vi "Export Origin - IV.vi"(8 "Error In":errorcluster, 9 "Workspace":path, 10 "Session properties":T4, 11 "IV measurement":T1={"Name"="", "Comment"="", "Time"=timestamp(0 s since 1904-01-01), "Folder"=path "", "IV properties"={"T"=0.0, "Vstart"=-0.5, "Vstop"=0.5, "Vpoints"=10.0, "Settling"=0.01, "I limit"=0.1, "Log mapping"=FALSE, "Averaging"=0.0}, "GUID"=""} {"IV properties"."Settling" min=0.0 max=65535.0}) -> (0 "Error Out":errorcluster)   [LabVIEW 2019]
doc: "Handles export of a I-V measurement to an Origin project, displays a GUI window"
uses:
  Type defs/Session properties Type Def.ctl
  Type defs/IV measurement Type Def.ctl
  Type defs/IV properties Type Def.ctl
  <vilib>/Utility/sysdir.llb/System Directory Type.ctl
panel:
  in  "Comment":T3(array[ring])=[enum."Temperature"] caption="Parameters to be placed in comments"
  in  "Save and exit after export":bool
  in  "Export to current Origin instance":bool
  out "String":string
  in  "Path":path caption="Export file as:"
  in  "Export":bool
  in  "Cancel":bool
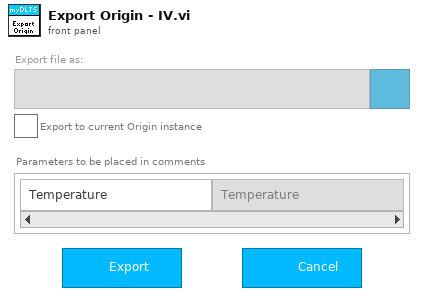
[diagram p1: front panel]
types:
  T1 = typedef "IV measurement Type Def.ctl" = cluster{"Name":string, "Comment":string, "Time":timestamp, "Folder":path, "IV properties":T2, "GUID":string}
  T2 = typedef "IV properties Type Def.ctl" = cluster{"T":dbl[unit], "Vstart":dbl[unit], "Vstop":dbl[unit], "Vpoints":dbl, "Settling":dbl[unit], "I limit":dbl[unit], "Log mapping":bool, "Averaging":dbl}
  T3 = enum16{"Temperature", "Settling", "Current limit"}[]
  T4 = typedef "Session properties Type Def.ctl" = cluster{"Session name":string, "Comment":string, "User":string, "Software version":dbl, "Created":timestamp, "Modified":timestamp, "Binary":bool, "GUID":string}
  T5 = enum32{"existing file", "new file", "new or existing file", "existing dir", "new dir", "new or existing dir", "existing file (use LLBs)", "new file (use LLBs)", "new or existing file (use LLBs)", "new or existing file or directory (use LLBs)", "existing dir (use LLBs)", "new dir (use LLBs)", "new or existing dir (use LLBs)", "existing file or dir", "new file or dir", "new or existing file or dir", "existing file or dir (use LLBs)", "new file or dir (use LLBs)"}
  T6 = typedef "System Directory Type.ctl" = i32
  T7 = enum8{"Enabled", "Disabled", "Disabled and Grayed Out"}
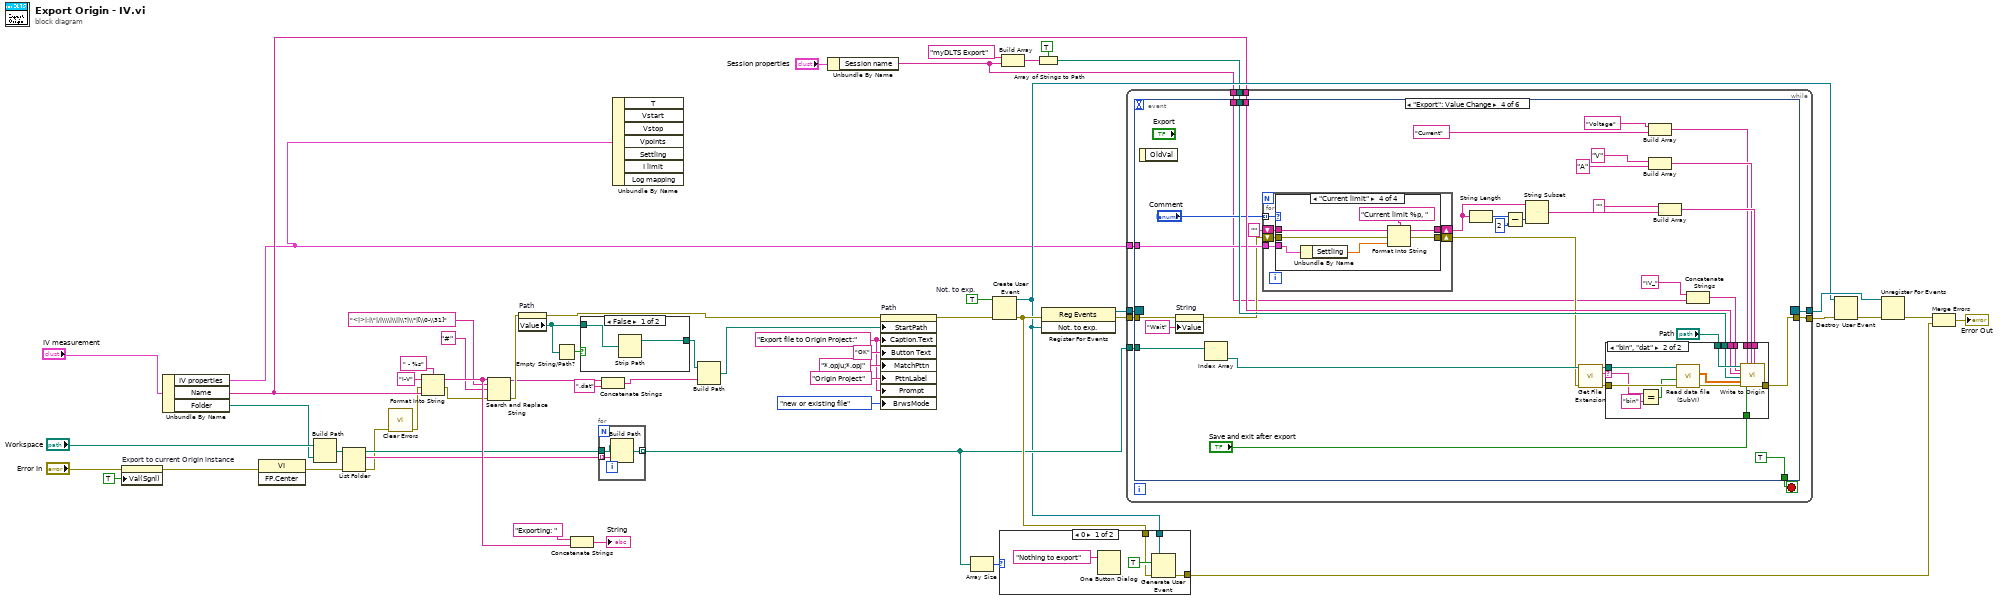
[diagram p0: block diagram]
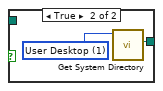
[diagram p2: hidden frame]
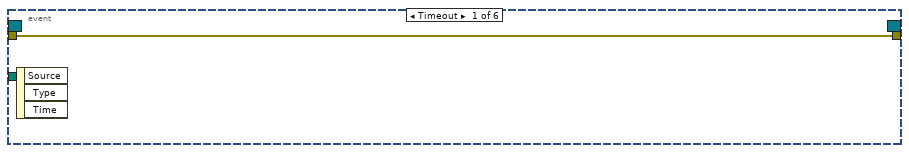
[diagram p4: hidden frame]
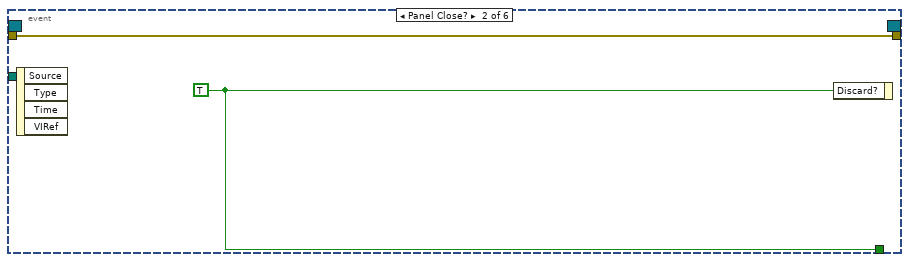
[diagram p5: hidden frame]
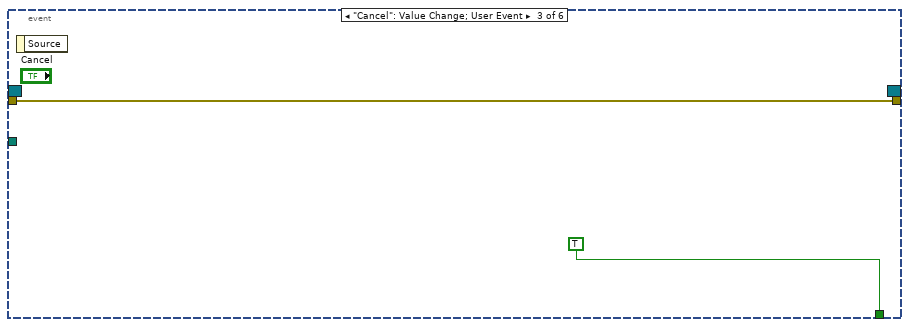
[diagram p6: hidden frame]
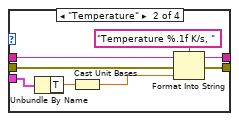
[diagram p8: hidden frame]
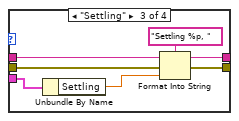
[diagram p9: hidden frame]
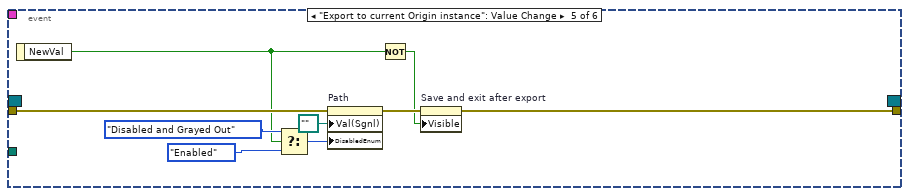
[diagram p11: hidden frame]
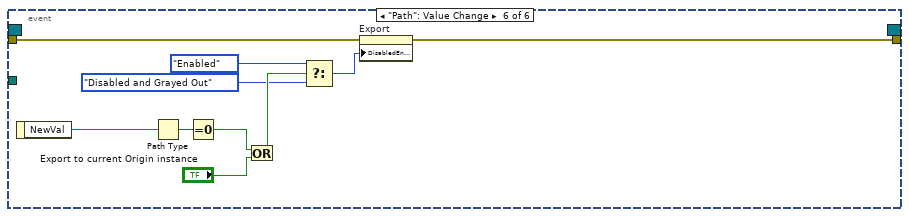
[diagram p12: hidden frame]
diagram:
  w27 = "Export file to Origin Project:"
  w54 = TRUE  # Not. to exp.
  n1 = property on="Export to current Origin instance" class="Bool (strict)"(error in="Error In", "Val(Sgnl)"=TRUE ("Value (Signaling)")) -> (error out=w6:errorcluster)  [unwired: 1 in, 1 out]
  n2 = Unbundle By Name("IV measurement") -> ("IV properties"=w4:T2, "Name"=w14:string, "Folder"=w32:path)
  n3 = invoke class="VI" method="FP.Center"(error in=w6) -> (error out=w16:errorcluster)  [unwired: 2 in, 2 out]
  n4 = Build Path(base path="Workspace", name or relative path=w32) -> (appended path=w25:path)
  n5 = List Folder(path=w25, error in=w16) -> (path out=w24:path, filenames=w31:string[], error out=w20:errorcluster)  [unwired: 2 in, 1 out]
  n6 = call <vilib>:"Clear Errors.vi"("error in (no error)"=w20) -> ("error out"=w2:errorcluster)  [unwired: 5 in, 1 out]
  n7 = Format Into String(format string=" - %s", initial string="I-V", error in=w2, w14) -> (resulting string=w43:string, error out=w19:errorcluster)
  n8 = Search and Replace String(input string=w43, search string="<|>|:|\"|/|\\\\|\\||\\?|\\*|[\\0-\\31]", replace string="#" ("replace string (\"\")"), error in=w19) -> (result string=w18:string, error out=w21:errorcluster)  [unwired: 4 in, 2 out]
  n9 = property on="Path" class="Path"(error in=w21) -> (error out=w33:errorcluster, "Value"=w39:path)  [unwired: 1 in, 1 out]
  n10 = Empty String/Path?(string/path=w39) -> (empty?=w40:bool)
  n11 = Concatenate Strings("Exporting: " ("string"), w43) -> (→"String":string)
  n12 = case shown="False" w40 {
    tunnel: w39 -> [w58 _]
    tunnel: [w57 w59] -> w35
    frame False {
      n13 = Strip Path(path=w58) -> (stripped path=w57:path)  [unwired: 1 out]
    }
    frame True {
      w60 = T6 1 items=["User Home"=0, "User Desktop"=1, "User Documents"=2, "User Application Data"=3, "User Preferences"=4, "User Temporary"=5, "Public Documents"=6, "Public Application Data"=7, "Public Preferences"=8, "Public Cache"=13, "System Core Libraries"=9, "System Installed Libraries"=10, "Application Files"=11, "Boot Volume Root"=12] ("system directory type")
      n14 = call <vilib>:"Get System Directory.vi"("system directory type"=w60) -> ("system directory"=w59:path)  [unwired: 10 in]
    }
  }
  n15 = for {
    tunnel: w24 -> [w63]
    tunnel: [w62] -> w49 mode=indexing
    tunnel: w31 -> [w61] mode=indexing
    n16 = Build Path(base path=w63, name or relative path=w61) -> (appended path=w62:path)
  }
  n17 = Concatenate Strings(w18, ".dat" ("string")) -> (w22:string)
  n18 = Unbundle By Name(w4) -> ()  [unwired: 7 out]
  n19 = Build Path(base path=w35, name or relative path=w22) -> (appended path=w34:path)
  n20 = Unbundle By Name("Session properties") -> ("Session name"=w3:string)
  n21 = property on="Path" class="Path"(error in=w33, "StartPath"=w34, "Caption.Text"=w27, "Button Text"="OK", "MatchPttn"="*.opju;*.opj", "PttnLabel"="Origin Project", "Prompt"=w27, "BrwsMode"=T5."new or existing file" ("Browse Options:Selection Mode")) -> (error out=w51:errorcluster)  [unwired: 1 in, 1 out]
  n22 = Array Size(array=w49) -> (size(s)=w55:i32)
  n23 = Create User Event(user event datatype=w54, error in=w51) -> (user event=w15:refnum<user-event>, error out=w50:errorcluster)
  n24 = case shown="0" w55 {
    tunnel: w15 -> [w67 _]
    tunnel: w50 -> [w65 w69]
    tunnel: [w64 w69] -> w44
    frame 0 {
      n25 = One Button Dialog(message="Nothing to export") -> ()  [unwired: 1 in, 1 out]
      n26 = Generate User Event(user event=w67, event data cluster=TRUE ("event data"), error in=w65) -> (error out=w64:errorcluster)  [unwired: 1 in, 1 out]
    }
    frame Default {
    }
  }
  n27 = Build Array("myDLTS Export" ("element"), w3) -> (w10:string[])
  n28 = Array of Strings to Path(0:w10, 1:TRUE ("relative")) -> (2:w9:path)
  n29 = register-events(error in=w50, w15) -> (reference out=w52:refnum<event-registration>, error out=w53:errorcluster)  [unwired: 1 in]
  n30 = while {
    tunnel: w53 -> [w79]
    tunnel: w49 -> [w77]
    tunnel: w52 -> [w76]
    tunnel: [w75] -> w47
    tunnel: w14 -> [w74]
    tunnel: w9 -> [w73]
    tunnel: [w72] -> w8
    tunnel: w4 -> [w71]
    tunnel: w3 -> [w70]
    stop <- w78 stop-if-true
    n31 = event shown="[3] \"Export\": Value Change" {
      selector: w76 -> [_ _ _ _ _ _]
      dyn-events: [_ _ _ _ _ _] -> w75
      timeout: _ -> [_ _ _ _ _ _]
      tunnel: w79 -> [w80 w81 w83 w113 w173 w180]
      tunnel: [w80 w81 w83 w116 w166 w175] -> w72
      tunnel: [_ w82 TRUE ("Discard?") TRUE _ _] -> w78
      tunnel: w77 -> [_ _ _ w118 _ _]
      tunnel: w74 -> [_ _ _ w111 _ _]
      tunnel: w73 -> [_ _ _ w110 _ _]
      tunnel: w71 -> [_ _ _ w96 _ _]
      tunnel: w70 -> [_ _ _ w85 _ _]
      event Timeout {
        n32 = event-data() -> ()  [unwired: 1 in, 3 out]
      }
      event Panel Close? {
        w82 = TRUE ("Discard?")
        n33 = event-data() -> ()  [unwired: 1 in, 4 out]
        n34 = event-data("Discard?"=w82) -> ()  [unwired: 1 in, 1 out]
      }
      event "Cancel": Value Change; User Event {
        n35 = event-data() -> ()  [unwired: 1 in, 1 out]
      }
      event "Export": Value Change {
        n36 = event-data() -> ()  [unwired: 1 in, 1 out]
        n37 = property on="String" class="Str"(error in=w113, "Value"="Wait" ("String")) -> (error out=w95:errorcluster)  [unwired: 1 in, 1 out]
        n38 = Index Array(array=w118) -> (element=w106:path)  [unwired: 1 in]
        n39 = for {
          tunnel: "Comment" -> [w124] mode=indexing
          tunnel: w96 -> [w123]
          shift-right: [w122] -> w94
          shift-left: w95 -> [w121]
          shift-right: [w120] -> w92
          shift-left: "" -> [w119]
          n40 = case shown="\"Current limit\"" w124 {
            tunnel: w123 -> [_ w130 w135 w142]
            tunnel: [w125 w134 w139 w146] -> w122
            tunnel: w121 -> [w125 w132 w137 w144]
            tunnel: [w126 w133 w138 w145] -> w120
            tunnel: w119 -> [w126 w131 w136 w143]
            frame Default {
            }
            frame "Temperature" {
              n41 = Unbundle By Name(w130) -> ("T"=w129:dbl[unit])
              n42 = Cast Unit Bases(0:w129) -> (2:w127:dbl)  [unwired: 1 in]
              n43 = Format Into String(format string="Temperature %.1f K/s, ", initial string=w131, error in=w132, w127) -> (resulting string=w133:string, error out=w134:errorcluster)
            }
            frame "Settling" {
              n44 = Unbundle By Name(w135) -> ("Settling"=w140:dbl[unit])
              n45 = Format Into String(format string="Settling %p, ", initial string=w136, error in=w137, w140) -> (resulting string=w138:string, error out=w139:errorcluster)
            }
            frame "Current limit" {
              n46 = Unbundle By Name(w142) -> ("Settling"=w147:dbl[unit])
              n47 = Format Into String(format string="Current limit %p, ", initial string=w143, error in=w144, w147) -> (resulting string=w145:string, error out=w146:errorcluster)
            }
          }
        }
        n48 = String Length(string=w92) -> (length=w91:i32)
        n49 = Subtract(x=w91, y=2) -> (x-y=w90:i32)
        n50 = String Subset(string=w92, length (rest)=w90) -> (substring=w88:string)  [unwired: 1 in]
        n51 = call <vilib>:"Get File Extension.vi"("error in (no error)"=w94, "file"=w106) -> ("error out"=w108:errorcluster, "lowercase file extension"=w107:string, "dup file"=w109:path)  [unwired: 5 in, 2 out]
        n52 = Build Array("Voltage", "Current") -> (w97:string[])
        n53 = Build Array("V", "A") -> (w98:string[])
        n54 = Build Array("", w88) -> (w99:string[])
        n55 = Concatenate Strings("IV_" ("Book name"), w85) -> (w86:string)
        n56 = case shown="\"bin\", \"dat\"" w107 {
          selector: w107 -> [_ w150]
          tunnel: w109 -> [_ w164]
          tunnel: w108 -> [w149 w163]
          tunnel: "Path" -> [_ w159]
          tunnel: w97 -> [_ w158]
          tunnel: w98 -> [_ w157]
          tunnel: w99 -> [_ w156]
          tunnel: [w149 w155] -> w116
          tunnel: "Save and exit after export" -> [_ w154]
          tunnel: w86 -> [_ w153]
          tunnel: w111 -> [_ w152]
          tunnel: w110 -> [_ w151]
          frame "False", Default {
          }
          frame "bin", "dat" {
            n57 = Equal?(x=w150, y="bin") -> (x = y?=w162:bool)
            n58 = call "Read data file (SubVI).vi"("error in"=w163, "Binary"=w162, "file path in"=w164) -> ("error out"=w160:errorcluster, "2D data"=w161:dbl[][])  [unwired: 6 in, 1 out]
            n59 = call "Write to Origin.vi"("Origin Project Path"=w159, "Book name"=w153, "Sheet name"=w152, "Folder name"=w151, "Data"=w161, "error in (no error)"=w160, "Column name"=w158, "Save and exit"=w154, "Column unit"=w157, "Column comment"=w156) -> ("error out"=w155:errorcluster)  [unwired: 9 in]
          }
        }
      }
      event "Export to current Origin instance": Value Change {
        n60 = event-data() -> ("NewVal"=w168:bool)  [unwired: 1 in]
        n61 = Select(t=T7."Disabled and Grayed Out" ("Disabled"), s=w168, f=T7."Enabled" ("Disabled")) -> (s? t:f=w169:T7)
        n62 = property on="Path" class="Path"(error in=w173, "Val(Sgnl)"=path "" ("Value (Signaling)"), "DisabledEnum"=w169) -> (error out=w172:errorcluster)  [unwired: 1 in, 1 out]
        n63 = Not(x=w168) -> (.not. x?=w167:bool)
        n64 = property on="Save and exit after export" class="Bool (strict)"(error in=w172, "Visible"=w167) -> (error out=w166:errorcluster)  [unwired: 1 in, 1 out]
      }
      event "Path": Value Change {
        n65 = event-data() -> ("NewVal"=w184:path)  [unwired: 1 in]
        n66 = Path Type(1:w184) -> (0:w183:i16)
        n67 = Equal To 0?(x=w183) -> (x = 0?=w181:bool)
        n68 = Or(x=w181, y="Export to current Origin instance") -> (x .or. y?=w179:bool)
        n69 = Select(t=T7."Enabled" ("Disabled"), s=w179, f=T7."Disabled and Grayed Out") -> (s? t:f=w178:T7)
        n70 = property on="Export" class="Bool"(error in=w180, "DisabledEnum"=w178) -> (error out=w175:errorcluster)  [unwired: 1 in, 1 out]
      }
    }
  }
  n71 = Destroy User Event(user event=w15, error in=w8) -> (error out=w48:errorcluster)
  n72 = Unregister For Events(event registration refnum=w47, error in=w48) -> (error out=w46:errorcluster)
  n73 = Merge Errors(w46, w44) -> (→"Error Out":errorcluster)
